vi "Smooth.vi"(10 "SPAN":i32, 11 "S":dbl[](array[numeric])) -> (3 "S_smooth":dbl[](array[numeric]))   [LabVIEW 2015, in "Digital Signal Processing.lvlib"]
uses:
  Digital Signal Processing.lvlib
  <vilib>/Analysis/baseanly.llb/Mean (DBL).vi
  <vilib>/Analysis/NI_AALBase.lvlib
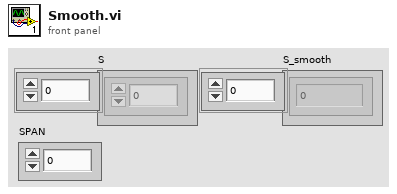
[diagram p1: front panel]
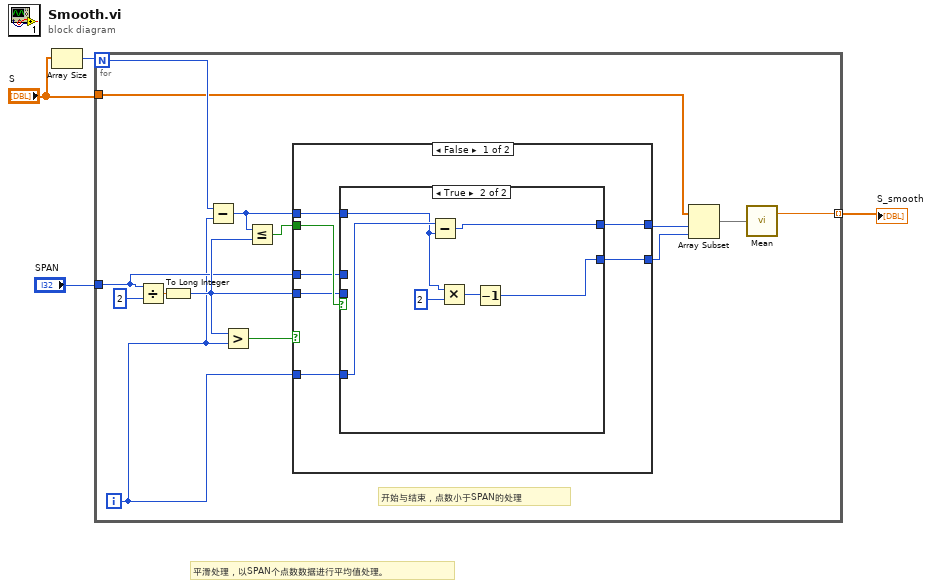
[diagram p0: block diagram]
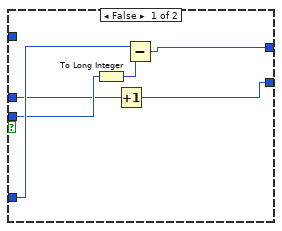
[diagram p2: hidden frame]
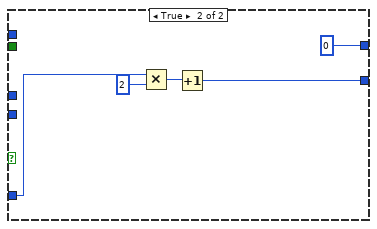
[diagram p3: hidden frame]
diagram:
  # "平滑处理，以SPAN个点数数据进行平均值处理。"
  n1 = Array Size(array="S") -> (size(s)=w3:i32)
  n2 = for {
    N: w3 -> [w18]
    tunnel: "S" -> [w12]
    tunnel: "SPAN" -> [w6]
    tunnel: [w10] -> w1 mode=indexing
    i -> [w5]
    # "开始与结束，点数小于SPAN的处理"
    n3 = Divide(x=w6, y=2) -> (x/y=w8:dbl)
    n4 = To Long Integer(number=w8) -> (32bit integer=w7:i32)
    n5 = Subtract(x=w18, y=w5) -> (x-y=w15:i32)
    n6 = Greater?(x=w7, y=w5) -> (0:w17:bool)
    n7 = Less Or Equal?(x=w15, y=w7) -> (x <= y?=w16:bool)
    n8 = case shown="False" w17 {
      tunnel: [w22 0] -> w14
      tunnel: w5 -> [w24 w41]
      tunnel: w16 -> [w25 _]
      tunnel: [w21 w38] -> w13
      tunnel: w15 -> [w23 _]
      tunnel: w7 -> [w20 _]
      tunnel: w6 -> [w19 _]
      frame False {
        n9 = case shown="True" w25 {
          tunnel: w24 -> [w31 w37]
          tunnel: w23 -> [_ w33]
          tunnel: [w29 w36] -> w22
          tunnel: [w28 w32] -> w21
          tunnel: w20 -> [w27 _]
          tunnel: w19 -> [w26 _]
          frame False {
            n10 = To Long Integer(number=w27) -> (32bit integer=w30:i32)
            n11 = Increment(x=w26) -> (x+1=w28:i32)
            n12 = Subtract(x=w31, y=w30) -> (x-y=w29:i32)
          }
          frame True {
            n13 = Subtract(x=w37, y=w33) -> (x-y=w36:i32)
            n14 = Multiply(x=w33, y=2) -> (x*y=w34:i32)
            n15 = Decrement(x=w34) -> (x-1=w32:i32)
          }
        }
      }
      frame True {
        n16 = Multiply(x=w41, y=2) -> (x*y=w39:i32)
        n17 = Increment(x=w39) -> (x+1=w38:i32)
      }
    }
    n18 = Array Subset(array=w12, index=w14, length=w13) -> (w11:dbl[])
    n19 = call-poly <vilib>:"Mean.vi"("X"=w11) -> ("mean"=w10:dbl)  [unwired: 1 out]
  }
  "S_smooth" <- w1
